vi "ILabVIEWItemProbe.vi"(11 "ILabVIEWItem":refnum<class "ILabVIEWItem.lvclass">) -> (2 "Value String":string, 3 "Boolean":bool)   [LabVIEW 2020, in "LabVIEWObjectInterfaces.lvlib" / "ILabVIEWItem.lvclass"]
uses:
  ILabVIEWItem.lvclass
panel:
  in  "Class type condition":string
  in  "Qualified name condition":string
  in  "Path condition":string
  out "Class type":string
  out "References":i32(listbox)
  out "Contained":i32(listbox)
  out "Qualified name":string
  out "Path":string
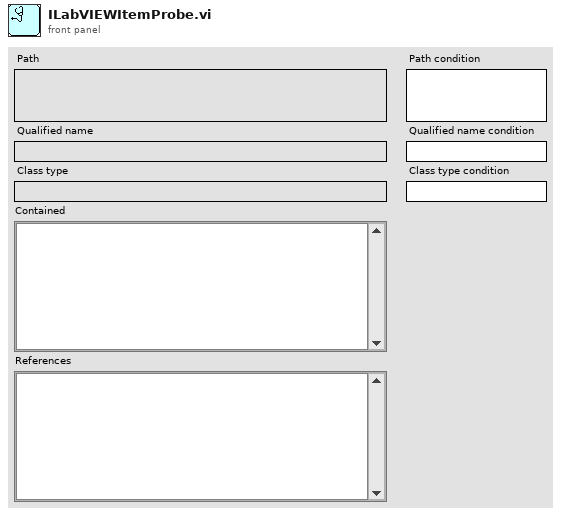
[diagram p1: front panel]
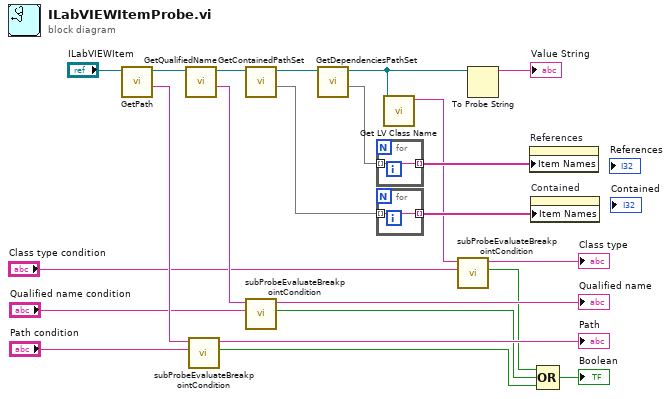
[diagram p0: block diagram]
diagram:
  n1 = call-dynamic "GetPath.vi"("ILabVIEWItem in"="ILabVIEWItem") -> ("Path"=w12:string, "ILabVIEWItem out"=w19:refnum<class "ILabVIEWItem.lvclass">)  [unwired: 8 in, 1 out]
  n2 = call-dynamic "GetQualifiedName.vi"("ILabVIEWItem in"=w19) -> ("Qualified name"=w10:string, "ILabVIEWItem out"=w22:refnum<class "ILabVIEWItem.lvclass">)  [unwired: 8 in, 1 out]
  n3 = call "subProbeEvaluateBreakpointCondition.vi"("String condition"="Path condition", "String in"=w12) -> ("Break?"=w2:bool, "String"=→"Path":string)  [unwired: 8 in]
  n4 = call-dynamic "GetContainedPathSet.vi"("ILabVIEWItem in"=w22) -> ("Contained"=w18:set{string}, "ILabVIEWItem out"=w21:refnum<class "ILabVIEWItem.lvclass">)  [unwired: 8 in, 1 out]
  n5 = call "subProbeEvaluateBreakpointCondition.vi"("String condition"="Qualified name condition", "String in"=w10) -> ("Break?"=w3:bool, "String"=→"Qualified name":string)  [unwired: 8 in]
  n6 = call-dynamic "GetDependenciesPathSet.vi"("ILabVIEWItem in"=w21) -> ("Dependencies"=w16:set{string}, "ILabVIEWItem out"=w14:refnum<class "ILabVIEWItem.lvclass">)  [unwired: 8 in, 1 out]
  n7 = for {
    tunnel: w16 -> [w24] mode=indexing
    tunnel: [w24] -> w15 mode=indexing
  }
  n8 = for {
    tunnel: w18 -> [w25] mode=indexing
    tunnel: [w25] -> w17 mode=indexing
  }
  n9 = call <vilib>:"Get LV Class Name.vi"("object"=w14) -> ("class name"=w7:string)  [unwired: 9 in, 1 out]
  n10 = call "subProbeEvaluateBreakpointCondition.vi"("String condition"="Class type condition", "String in"=w7) -> ("Break?"=w4:bool, "String"=→"Class type":string)  [unwired: 8 in]
  n11 = To Probe String(7:w14) -> (3:→"Value String":string)  [unwired: 2 in, 1 out]
  n12 = property on="References" class="LstBox (strict)"("Item Names"=w15) -> ()  [unwired: 2 in, 2 out]
  n13 = property on="Contained" class="LstBox (strict)"("Item Names"=w17) -> ()  [unwired: 2 in, 2 out]
  n14 = Compound Arithmetic op=OR(w4, w3, w2) -> (→"Boolean":bool)
